vi "探头窗口-35-5列7行.vi"   [LabVIEW 2013]
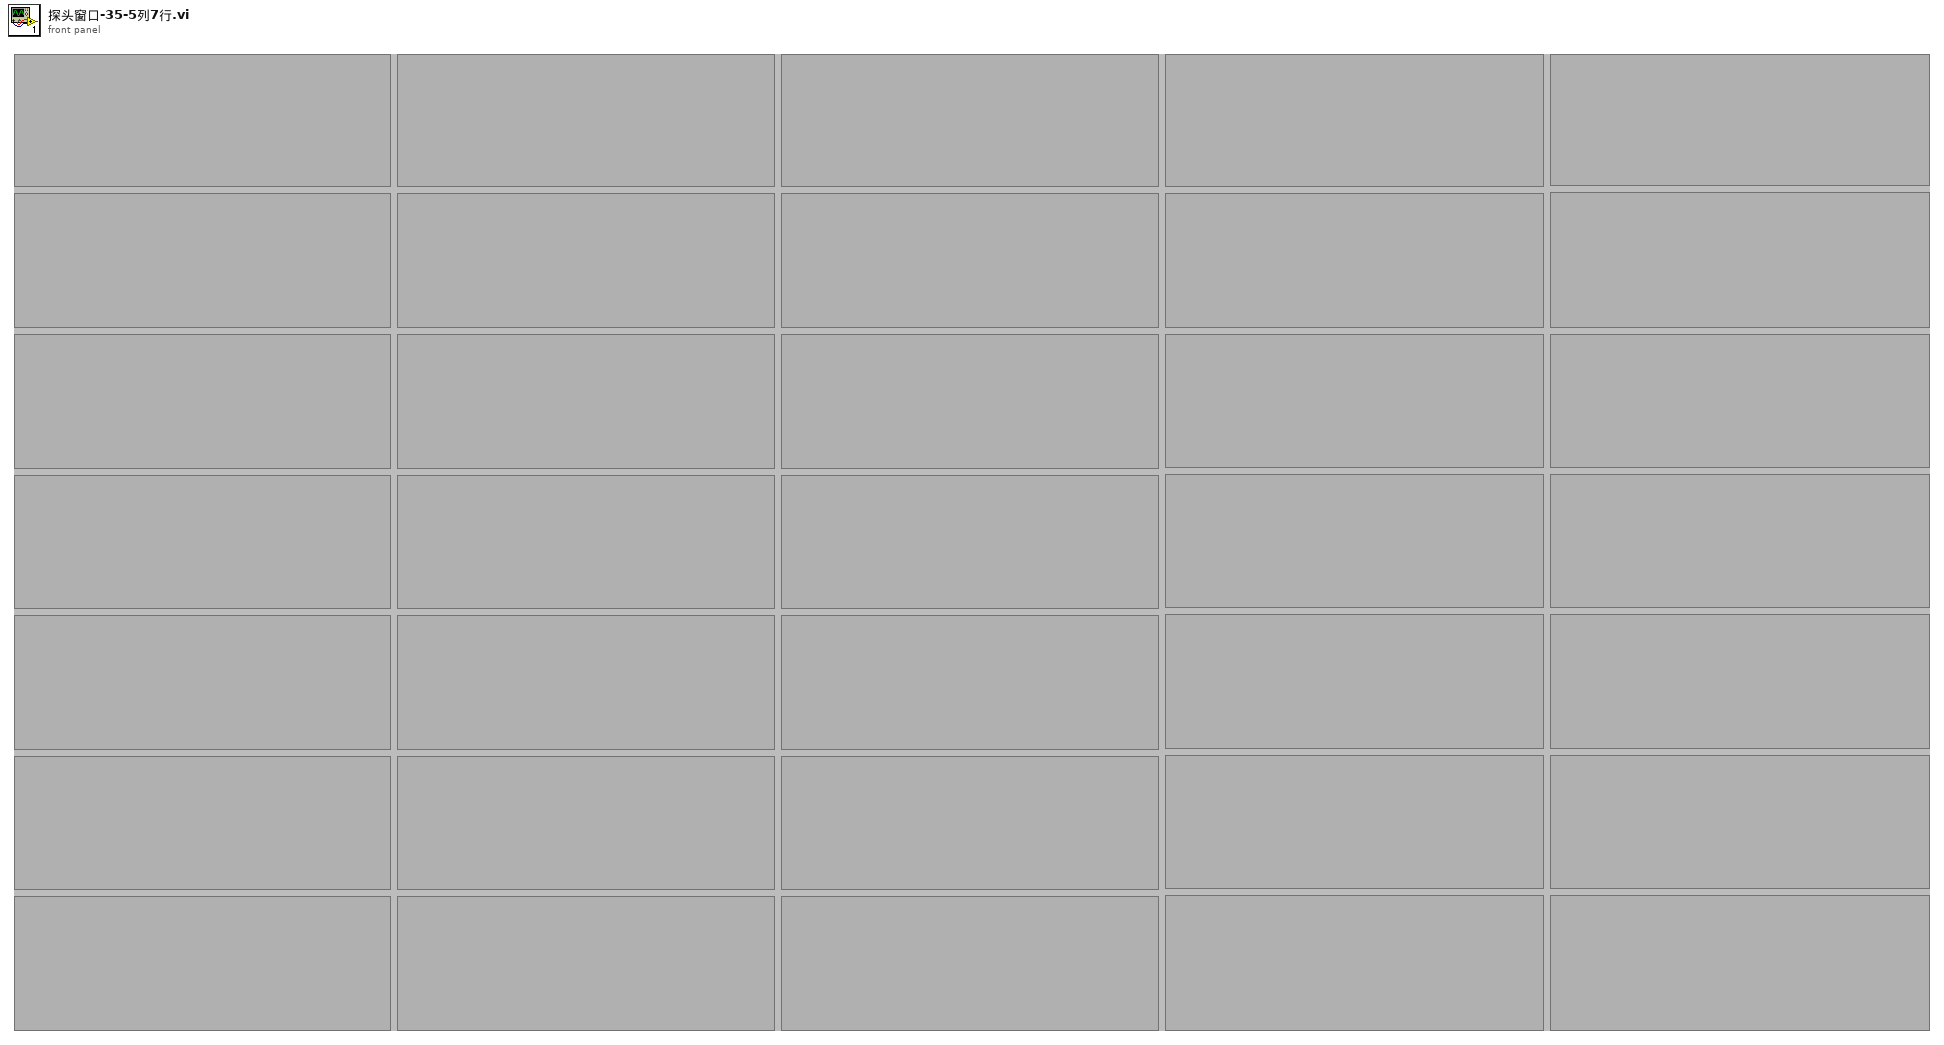
[diagram p1: front panel]
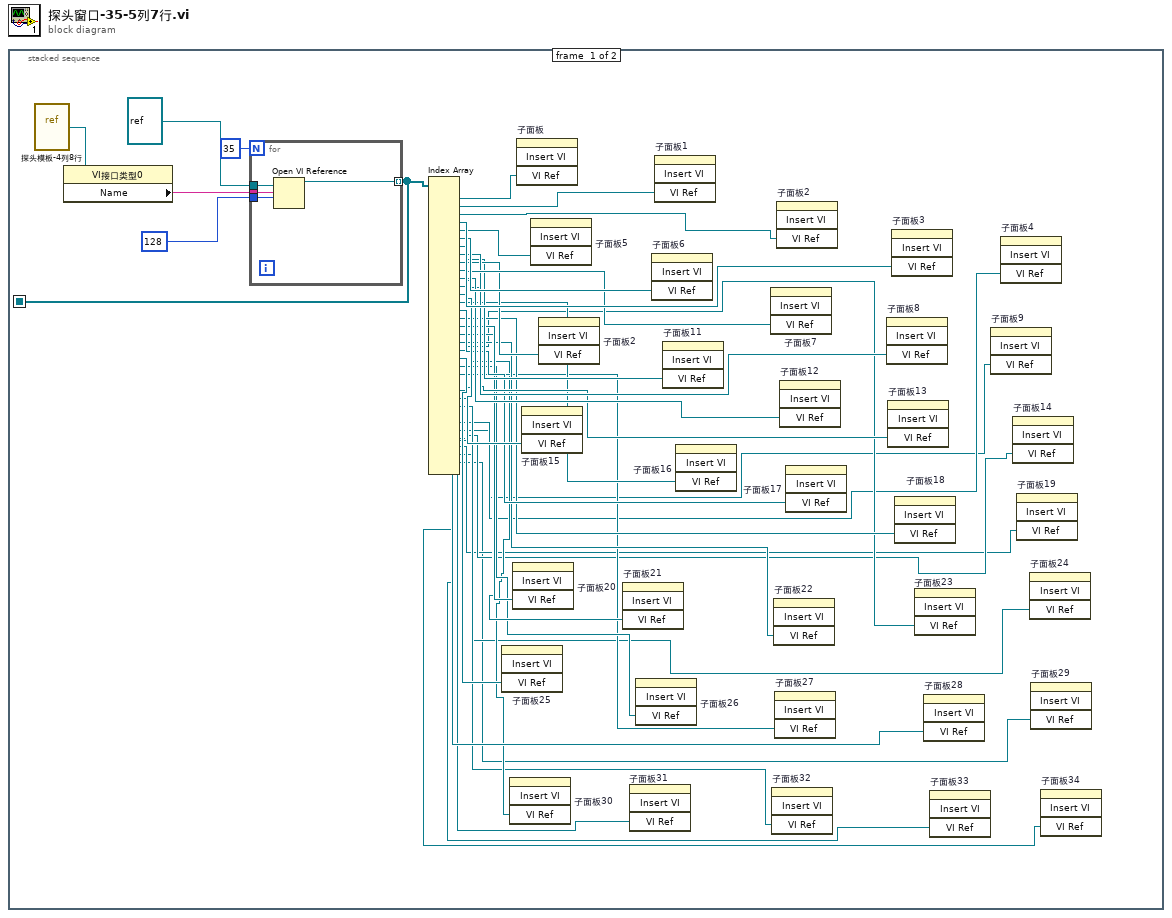
[diagram p0: block diagram]
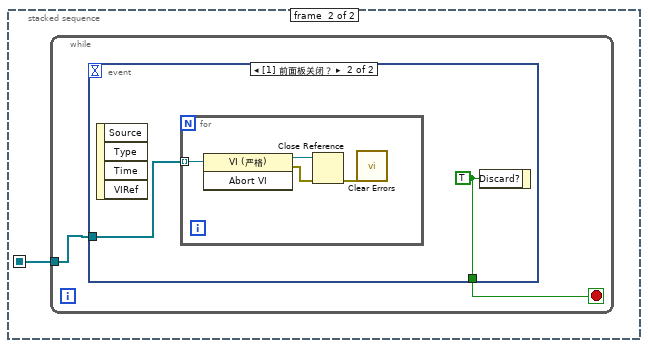
[diagram p2: hidden frame]
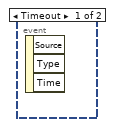
[diagram p3: hidden frame]
diagram:
  n1 = stacked-sequence {
    seq-local: [w36 _] -> [_ w46]
    frame #0 {
      n2 = vi-ref "探头模板-4列8行.vi"() -> (w41:refnum<vi>)
      n3 = property class="VI接口类型0"(reference=w41) -> ("Name"=w40:string)  [unwired: 1 in, 2 out]
      n4 = for {
        N: 35 -> [_]
        tunnel: w40 -> [w45]
        tunnel: 128 ("选项") -> [w44]
        tunnel: refnum<vi> refnum ("类型说明符VI引用句柄（仅用于类型）") -> [w43]
        tunnel: [w42] -> w36 mode=indexing
        n5 = Open VI Reference(type specifier VI Refnum (for type only)=w43, vi path=w45, options=w44) -> (vi reference=w42:refnum<vi>)  [unwired: 3 in, 1 out]
      }
      n6 = Index Array(array=w36) -> (element #1=w35:refnum<vi>, element #2=w34:refnum<vi>, element #3=w33:refnum<vi>, element #4=w32:refnum<vi>, element #5=w31:refnum<vi>, element #6=w30:refnum<vi>, element #7=w29:refnum<vi>, element #8=w28:refnum<vi>, element #9=w27:refnum<vi>, element #10=w26:refnum<vi>, element #11=w25:refnum<vi>, element #12=w24:refnum<vi>, element #13=w23:refnum<vi>, element #14=w22:refnum<vi>, element #15=w21:refnum<vi>, element #16=w20:refnum<vi>, element #17=w19:refnum<vi>, element #18=w18:refnum<vi>, element #19=w17:refnum<vi>, element #20=w16:refnum<vi>, element #21=w15:refnum<vi>, element #22=w14:refnum<vi>, element #23=w13:refnum<vi>, element #24=w12:refnum<vi>, element #25=w11:refnum<vi>, element #26=w10:refnum<vi>, element #27=w9:refnum<vi>, element #28=w8:refnum<vi>, element #29=w7:refnum<vi>, element #30=w6:refnum<vi>, element #31=w5:refnum<vi>, element #32=w4:refnum<vi>, element #33=w3:refnum<vi>, element #34=w2:refnum<vi>, element #35=w1:refnum<vi>)  [unwired: 35 in]
      n7 = invoke on="子面板25" class="SubPnl" method="Insert VI"("VI Ref"=w15) -> ()  [unwired: 3 in, 4 out]
      n8 = invoke on="子面板30" class="SubPnl" method="Insert VI"("VI Ref"=w11) -> ()  [unwired: 3 in, 4 out]
      n9 = invoke on="子面板20" class="SubPnl" method="Insert VI"("VI Ref"=w19) -> ()  [unwired: 3 in, 4 out]
      n10 = invoke on="子面板" class="子面板" method="Insert VI"("VI Ref"=w35) -> ()  [unwired: 3 in, 4 out]
      n11 = invoke on="子面板15" class="SubPnl" method="Insert VI"("VI Ref"=w23) -> ()  [unwired: 3 in, 4 out]
      n12 = invoke on="子面板5" class="SubPnl" method="Insert VI"("VI Ref"=w31) -> ()  [unwired: 3 in, 4 out]
      n13 = invoke on="子面板2" class="SubPnl" method="Insert VI"("VI Ref"=w27) -> ()  [unwired: 3 in, 4 out]
      n14 = invoke on="子面板21" class="SubPnl" method="Insert VI"("VI Ref"=w18) -> ()  [unwired: 3 in, 4 out]
      n15 = invoke on="子面板31" class="SubPnl" method="Insert VI"("VI Ref"=w10) -> ()  [unwired: 3 in, 4 out]
      n16 = invoke on="子面板26" class="SubPnl" method="Insert VI"("VI Ref"=w14) -> ()  [unwired: 3 in, 4 out]
      n17 = invoke on="子面板6" class="SubPnl" method="Insert VI"("VI Ref"=w30) -> ()  [unwired: 3 in, 4 out]
      n18 = invoke on="子面板1" class="SubPnl" method="Insert VI"("VI Ref"=w34) -> ()  [unwired: 3 in, 4 out]
      n19 = invoke on="子面板11" class="SubPnl" method="Insert VI"("VI Ref"=w26) -> ()  [unwired: 3 in, 4 out]
      n20 = invoke on="子面板16" class="SubPnl" method="Insert VI"("VI Ref"=w22) -> ()  [unwired: 3 in, 4 out]
      n21 = invoke on="子面板7" class="SubPnl" method="Insert VI"("VI Ref"=w29) -> ()  [unwired: 3 in, 4 out]
      n22 = invoke on="子面板32" class="SubPnl" method="Insert VI"("VI Ref"=w9) -> ()  [unwired: 3 in, 4 out]
      n23 = invoke on="子面板22" class="SubPnl" method="Insert VI"("VI Ref"=w17) -> ()  [unwired: 3 in, 4 out]
      n24 = invoke on="子面板27" class="SubPnl" method="Insert VI"("VI Ref"=w13) -> ()  [unwired: 3 in, 4 out]
      n25 = invoke on="子面板2" class="SubPnl" method="Insert VI"("VI Ref"=w33) -> ()  [unwired: 3 in, 4 out]
      n26 = invoke on="子面板12" class="SubPnl" method="Insert VI"("VI Ref"=w25) -> ()  [unwired: 3 in, 4 out]
      n27 = invoke on="子面板17" class="SubPnl" method="Insert VI"("VI Ref"=w21) -> ()  [unwired: 3 in, 4 out]
      n28 = invoke on="子面板8" class="SubPnl" method="Insert VI"("VI Ref"=w28) -> ()  [unwired: 3 in, 4 out]
      n29 = invoke on="子面板13" class="SubPnl" method="Insert VI"("VI Ref"=w24) -> ()  [unwired: 3 in, 4 out]
      n30 = invoke on="子面板3" class="SubPnl" method="Insert VI"("VI Ref"=w32) -> ()  [unwired: 3 in, 4 out]
      n31 = invoke on="子面板18" class="SubPnl" method="Insert VI"("VI Ref"=w20) -> ()  [unwired: 3 in, 4 out]
      n32 = invoke on="子面板23" class="SubPnl" method="Insert VI"("VI Ref"=w16) -> ()  [unwired: 3 in, 4 out]
      n33 = invoke on="子面板28" class="SubPnl" method="Insert VI"("VI Ref"=w12) -> ()  [unwired: 3 in, 4 out]
      n34 = invoke on="子面板33" class="SubPnl" method="Insert VI"("VI Ref"=w8) -> ()  [unwired: 3 in, 4 out]
      n35 = invoke on="子面板9" class="SubPnl" method="Insert VI"("VI Ref"=w6) -> ()  [unwired: 3 in, 4 out]
      n36 = invoke on="子面板4" class="SubPnl" method="Insert VI"("VI Ref"=w7) -> ()  [unwired: 3 in, 4 out]
      n37 = invoke on="子面板14" class="SubPnl" method="Insert VI"("VI Ref"=w5) -> ()  [unwired: 3 in, 4 out]
      n38 = invoke on="子面板19" class="SubPnl" method="Insert VI"("VI Ref"=w4) -> ()  [unwired: 3 in, 4 out]
      n39 = invoke on="子面板24" class="SubPnl" method="Insert VI"("VI Ref"=w3) -> ()  [unwired: 3 in, 4 out]
      n40 = invoke on="子面板29" class="SubPnl" method="Insert VI"("VI Ref"=w2) -> ()  [unwired: 3 in, 4 out]
      n41 = invoke on="子面板34" class="SubPnl" method="Insert VI"("VI Ref"=w1) -> ()  [unwired: 3 in, 4 out]
    }
    frame #1 {
      n42 = while {
        tunnel: w46 -> [w47]
        stop <- w48 stop-if-true
        n43 = event shown="[1] 前面板关闭？" {
          selector: _ -> [_ _]
          dyn-events: _ -> [_ _]
          timeout: _ -> [_ _]
          tunnel: [_ w50] -> w48
          tunnel: w47 -> [_ w49]
          event Timeout {
            n44 = event-data() -> ()  [unwired: 1 in, 3 out]
          }
          event Panel Close? {
            w50 = TRUE ("放弃？")
            n45 = event-data() -> ()  [unwired: 1 in, 4 out]
            n46 = for {
              tunnel: w49 -> [w54] mode=indexing
              n47 = invoke class="VI (严格)" method="Abort VI"(reference=w54) -> (reference out=w52:refnum<vi>, error out=w53:errorcluster)  [unwired: 2 in, 1 out]
              n48 = Close Reference(reference=w52, error in (no error)=w53) -> (error out=w51:errorcluster)
              n49 = call <vilib>:"Clear Errors.vi"("error in (no error)"=w51) -> ()  [unwired: 6 in, 1 out]
            }
            n50 = event-data("Discard?"=w50) -> ()  [unwired: 1 in, 1 out]
          }
        }
      }
    }
  }
